vi "Set Image Current ROI.vi"(7 "Image Refnum":refnum<vi>, 8 "error in (no error)":errorcluster, 10 "Current ROI":i32, 11 "Stored ROIs in":T1[](array[typedef]) {"ROI Descriptor"."Contours"."Type" items=["No Selection", "Point", "Line", "Rectangle", "Oval", "Polygon", "Freehand Region", "Annulus", "Unused2", "Unused3", "Broken Line", "Freehand Line", "Rotated Rectangle"]}) -> (0 "Error Out":errorcluster)   [LabVIEW 2021, in "Image.lvlib"]
uses:
  Image.lvlib
  Named ROI Description.ctl
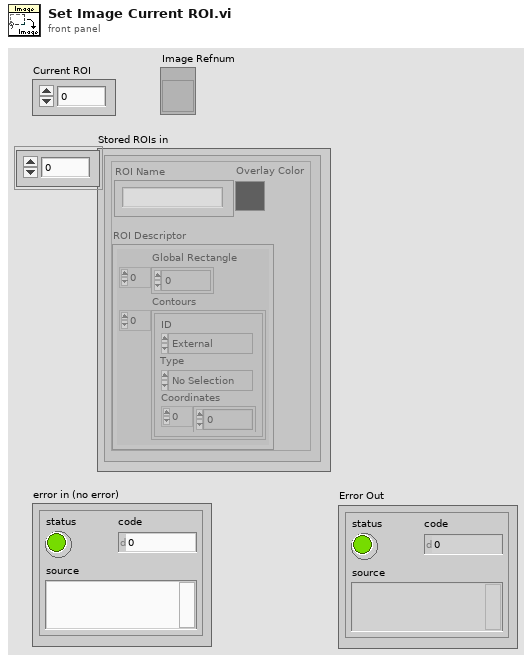
[diagram p1: front panel]
types:
  T1 = typedef "Image.lvlib/Named ROI Description.ctl" = cluster{"ROI Descriptor":T2, "ROI Name":string, "Overlay Color":u32}
  T2 = typedef "ROI Descriptor" = cluster{"Global Rectangle":i32[], "Contours":cluster{"ID":enum32{"External", "Internal"}, "Type":u32, "Coordinates":i32[]}[]}
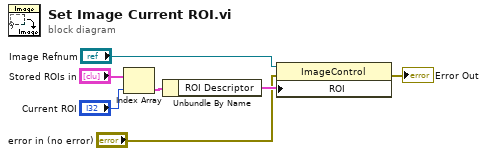
[diagram p0: block diagram]
diagram:
  n1 = Index Array(array="Stored ROIs in", index="Current ROI") -> (element=w3:T1)
  n2 = Unbundle By Name(w3) -> ("ROI Descriptor"=w2:T2)
  n3 = property class="ImageControl"(reference="Image Refnum", error in="error in (no error)", "ROI"=w2) -> (error out=→"Error Out":errorcluster)  [unwired: 1 out]
